vi "GetType.vi"(8 "error in (no error)":errorcluster, 11 "Configure FM Enabled [FM] Msg":refnum<class "Configure FM Enabled [FM] Msg.lvclass">) -> (0 "error out":errorcluster, 2 "Data Sample":variant, 3 "Configure FM Enabled [FM] Msg":refnum<class "Configure FM Enabled [FM] Msg.lvclass">)   [LabVIEW 2015, in "CS++Fgen.lvlib" / "Configure FM Enabled [FM] Msg.lvclass"]
doc: "This VI delivers a sample of the data type format the message expects."
uses:
  Configure FM Enabled [FM] Msg.lvclass
  Configure FM Enabled [FM] Msg.lvclass/Configure FM Enabled [FM] Msg.ctl
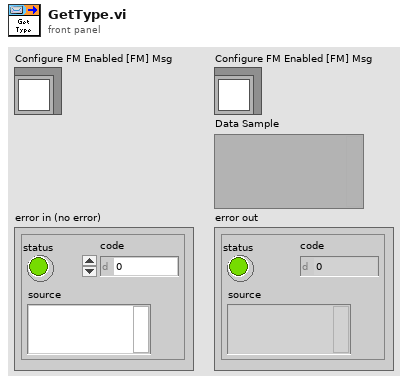
[diagram p1: front panel]
types:
  T1 = cluster{"Channel Name (\"\")":string, "FM enabled (True)":bool}
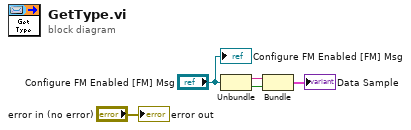
[diagram p0: block diagram]
diagram:
  n1 = Unbundle("Configure FM Enabled [FM] Msg") -> (w2:string, w1:bool)
  n2 = Bundle("Channel Name (\"\")"=w2, "FM enabled (True)"=w1) -> (→"Data Sample":T1)  [unwired: 1 in]
  "error out" <- "error in (no error)"
  "Configure FM Enabled [FM] Msg" <- "Configure FM Enabled [FM] Msg"
